vi "UnloadSession.vi"(7 "DLL Path":path, 8 "error in (no error)":errorcluster, 11 "session id in":i32) -> (0 "error out":errorcluster, 3 "session id out":i32)   [LabVIEW 2017, in "ONNX Class Library.lvlib"]
doc: "/**\n * @brief Выгрузить сессию из памяти (освободить веса модели)\n * \n * Эта функция освобождает память, занимаемую моделью (веса, вычислительный граф),\n * но сохраняет SessionID, путь к файлу и метаданные (имена входов/выходов, формы).\n * Позволяет временно освободить память и позже перезагрузить модель через ReloadSession.\n * \n * @param sessionId [IN] ID сессии для выгрузки\n * \n * @return int32: 0 при успешной выгрузке\n * @return int32: -1 если сессия не найдена\n * \n * @note Путь к модели сохраняется для возможности перезагрузки\n * @note SessionID остаётся валидным\n */\nint UnloadSession(int sessionId);"
uses:
  ONNX Class Library.lvlib
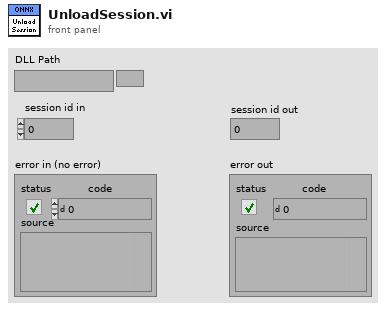
[diagram p1: front panel]
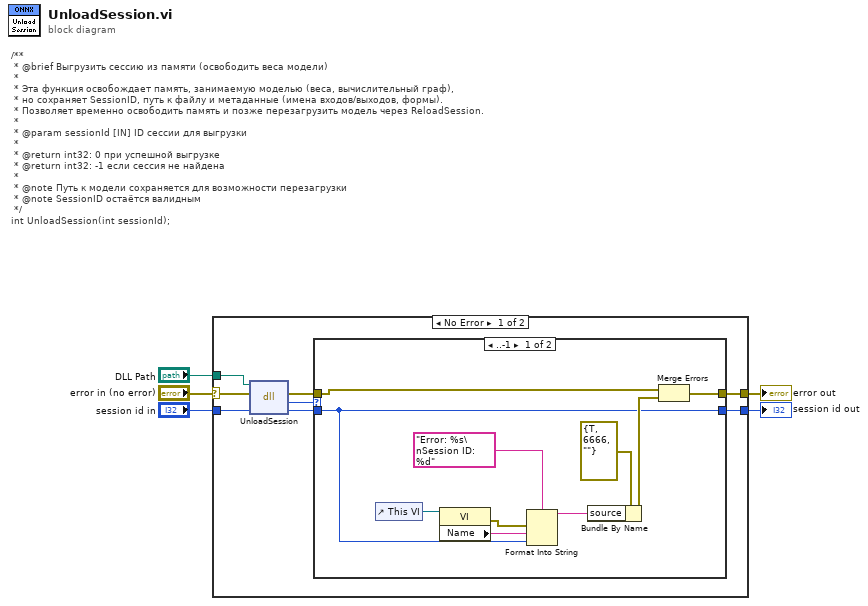
[diagram p0: block diagram]
diagram:
  # "/**\n * @brief Выгрузить сессию из памяти (освободить веса модели)\n * \n * Эта функция освобождает память, занимаемую моделью (веса, вычислительный граф),\n * но сохраняет SessionID, путь к файлу и метаданные (имена входов/выходов, формы).\n * Позволяет временно освободить память и позже перезагрузить модель через ReloadSession.\n * \n * @param sessionId [IN] ID сессии для выгрузки\n * \n * @return int32: 0 при успешной выгрузке\n * @return int32: -1 если сессия не найдена\n * \n * @note Путь к модели сохраняется для возможности перезагрузки\n * @note SessionID остаётся валидным\n */\nint UnloadSession(int sessionId);"
  n1 = case shown="No Error" "error in (no error)" {
    selector: "error in (no error)" -> [w7 w27]
    tunnel: "session id in" -> [w13 w26]
    tunnel: [w12 w27] -> w4
    tunnel: [w11 w26] -> w3
    tunnel: "DLL Path" -> [w6 _]
    frame No Error {
      n2 = dll-call lib="home/ivan/LabVIEWData/ONNX/Test/libonnx_wrapper/unix64/libonnx_wrapper.so" fn="UnloadSession"(path in=w6, error in=w7, "sessionId"=w13) -> (error out=w10:errorcluster, "return"=w9:i32, "sessionId"=w8:i32)  [unwired: 1 in, 1 out]
      n3 = case shown="..-1" w9 {
        tunnel: w10 -> [w14 w25]
        tunnel: [w15 w25] -> w12
        tunnel: w8 -> [w16 w24]
        tunnel: [w16 w24] -> w11
        frame ..-1 {
          n4 = control-ref of="This VI"() -> (w20:refnum<vi>)
          n5 = property class="VI"(reference=w20) -> (error out=w17:errorcluster, "Name"=w19:string)  [unwired: 1 in, 1 out]
          n6 = Format Into String(format string="Error: %s\nSession ID: %d", error in=w17, w19, w16) -> (resulting string=w21:string)  [unwired: 1 in, 1 out]
          n7 = Bundle By Name(cluster=errorcluster {"status"=TRUE, "code"=6666, "source"=""} ("error out"), "source"=w21) -> (w22:errorcluster)
          n8 = Merge Errors(w14, w22) -> (w15:errorcluster)
        }
        frame 0.. {
        }
      }
    }
    frame Error {
    }
  }
  "error out" <- w4
  "session id out" <- w3
